vi "仪器参数存表.vi"() -> ()   [LabVIEW 2016]
panel:
  out "error out":errorcluster
  out "columns":string[](array[string])
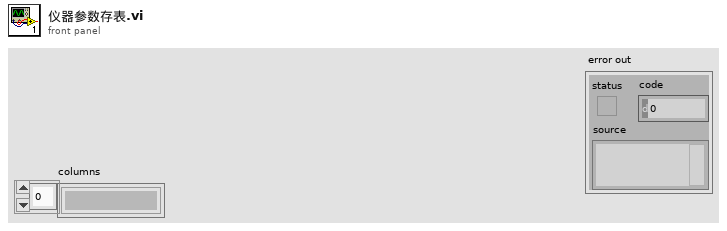
[diagram p1: front panel]
types:
  T1 = cluster{"测量量程":dbl, "测量精度":dbl, "测量间隔":dbl, "消解温度":dbl, "消解时长":dbl, "空白校准时间":timestamp, "曲线截距":dbl, "曲线斜率":dbl, "测量检出限":dbl, "测量信号值":dbl, "线性相关系数":dbl, "二次多项式系数":dbl, "标样校准时间":timestamp, "单位":enum16{"ug/L", "mg/L"}}
  T2 = cluster{"时间标识":timestamp, "仪器参数":string, "测量量程":dbl, "测量精度":dbl, "测量间隔":dbl, "消解温度":dbl, "消解时长":dbl, "空白校准时间":timestamp, "曲线截距":dbl, "曲线斜率":dbl, "测量检出限":dbl, "测量信号值":dbl, "线性相关系数":dbl, "二次多项式系数":dbl, "标样校准时间":timestamp, "单位":enum16{"ug/L", "mg/L"}}
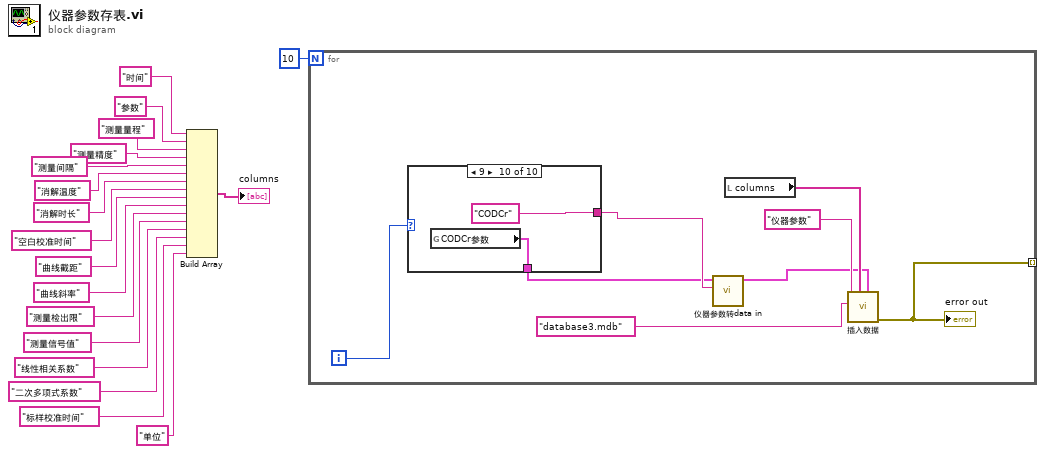
[diagram p0: block diagram]
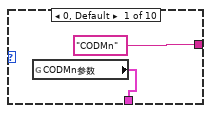
[diagram p2: hidden frame]
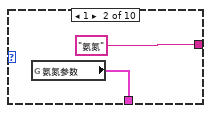
[diagram p3: hidden frame]
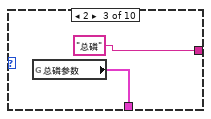
[diagram p4: hidden frame]
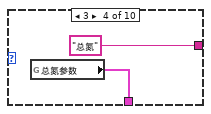
[diagram p5: hidden frame]
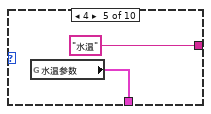
[diagram p6: hidden frame]
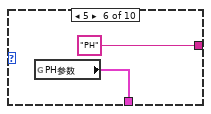
[diagram p7: hidden frame]
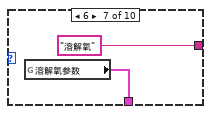
[diagram p8: hidden frame]
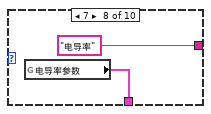
[diagram p9: hidden frame]
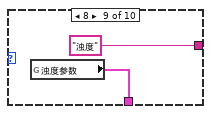
[diagram p10: hidden frame]
diagram:
  n1 = Build Array("时间" ("元素"), "参数" ("元素"), "测量量程", "测量精度" ("元素"), "测量间隔", "消解温度", "消解时长", "空白校准时间", "曲线截距", "曲线斜率", "测量检出限", "测量信号值", "线性相关系数", "二次多项式系数", "标样校准时间", "单位" ("元素")) -> (→"columns":string[])
  n2 = for {
    N: 10 -> [_]
    tunnel: [w23] -> _ mode=indexing
    i -> [w26]
    n3 = case shown="9" w26 {
      tunnel: [w27 w29 w31 w34 w36 w38 w40 w42 w44 w46] -> w19
      tunnel: ["CODMn" ("database") "氨氮" ("database") "总磷" ("database") "总氮" ("database") "水温" ("database") "PH" ("database") "溶解氧" ("database") "电导率" ("database") "浊度" ("database") "CODCr" ("database")] -> w22
      frame 0, Default {
        n4 = global read "在线监测仪器仪表参数.vi" "CODMn参数"() -> (w27:T1)
      }
      frame 1 {
        n5 = global read "在线监测仪器仪表参数.vi" "氨氮参数"() -> (w29:T1)
      }
      frame 2 {
        n6 = global read "在线监测仪器仪表参数.vi" "总磷参数"() -> (w31:T1)
      }
      frame 3 {
        n7 = global read "在线监测仪器仪表参数.vi" "总氮参数"() -> (w34:T1)
      }
      frame 4 {
        n8 = global read "在线监测仪器仪表参数.vi" "水温参数"() -> (w36:T1)
      }
      frame 5 {
        n9 = global read "在线监测仪器仪表参数.vi" "PH参数"() -> (w38:T1)
      }
      frame 6 {
        n10 = global read "在线监测仪器仪表参数.vi" "溶解氧参数"() -> (w40:T1)
      }
      frame 7 {
        n11 = global read "在线监测仪器仪表参数.vi" "电导率参数"() -> (w42:T1)
      }
      frame 8 {
        n12 = global read "在线监测仪器仪表参数.vi" "浊度参数"() -> (w44:T1)
      }
      frame 9 {
        n13 = global read "在线监测仪器仪表参数.vi" "CODCr参数"() -> (w46:T1)
      }
    }
    n14 = call "仪器参数转data in.vi"(10:"仪器参数"=w22, 11:"仪器参数"=w19) -> ("data in"=w20:T2)  [unwired: 9 in]
    n15 = local read "columns"() -> (w24:string[])
    n16 = call "插入数据.vi"("data"=w20, "columns"=w24, "database"="database3.mdb", "table"="仪器参数" ("database")) -> ("error out"=w23:errorcluster)  [unwired: 7 in]
    "error out" <- w23
  }
